vi "Acquisition Done.vi"(8 "error in (no error)":errorcluster, 11 "Abstract Camera in":refnum<class "Abstract Camera.lvclass">) -> (0 "error out":errorcluster, 2 "Acquisition Done":bool, 3 "Abstract Camera out":refnum<class "Abstract Camera.lvclass">)   [LabVIEW 2019, in "Abstract Camera.lvclass"]
uses:
  Abstract Camera.lvclass
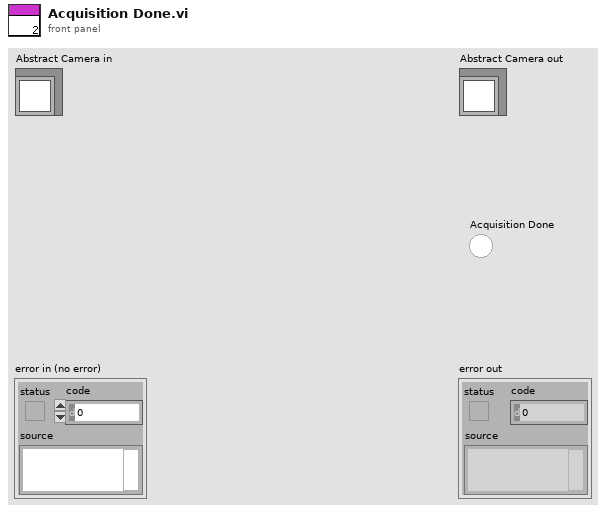
[diagram p1: front panel]
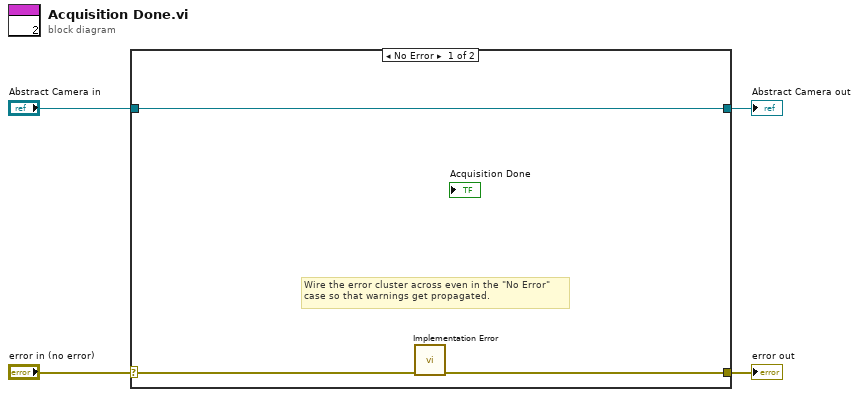
[diagram p0: block diagram]
diagram:
  n1 = case shown="No Error" "error in (no error)" {
    selector: "error in (no error)" -> [w6 w9]
    tunnel: [w5 w9] -> w3
    tunnel: [w7 w8] -> w1
    tunnel: "Abstract Camera in" -> [w7 w8]
    frame No Error {
      # "Wire the error cluster across even in the \"No Error\"\ncase so that warnings get propagated."
      n2 = call "Implementation Error.vi"("error in (no error)"=w6) -> ("error out"=w5:errorcluster)  [unwired: 10 in]
    }
    frame Error {
    }
  }
  "error out" <- w3
  "Abstract Camera out" <- w1
